vi "Intake Controller.vi"(8 "error in":errorcluster) -> ()   [LabVIEW 2019]
doc: "This VI executes continuously carrying out the current operation and responding to updates or new operations. It will often contain the timing or control code that is difficult to place directly in TeleOp. This VI generally opens all sensors and motors and isolates the rest of the robot code from knowing how the operations are carried out."
uses:
  <vilib>/Rock Robotics/WPI/Framework/Completion Status.ctl
  Intake Setpoints.ctl
  Intake Operations.ctl
  <vilib>/Rock Robotics/WPI/ThirdParty/REV Robotics/SPARK MAX/Typedef/Spark MAX Idle Mode.ctl
  <vilib>/Rock Robotics/WPI/ThirdParty/REV Robotics/SPARK MAX/Typedef/Spark MAX Control Type.ctl
  <vilib>/Rock Robotics/Network Tables/NT Write Boolean.vi
panel:
  out "Sensor Position":dbl
  out "up/down chart":T1(graph)
  in  "PID Constants":T2={"P Gain"=0.0325, "I Gain"=0.0, "D Gain"=0.0, "F Gain"=0.0, "I Zone"=0.0, "Min Output"=-0.3, "Max Output"=1.0}
  in  "Interactive Values":T3
  out "Current\nCmd":string
  in  "Buttons":cluster{"Execute Cmd":bool, "Abort Cmd":bool}
  out "Command Timing":cluster{"Start Time (ms)":u32, "Iterations":i32}
  out "Status":T5
  # "Tip: It may be helpful to observe inputs and sensor values.\nYou may also want to display tuning or debugging controls."
  # "Interactive Command: You may fill in the settings for a command\nand schedule it with the Execute button. You can observe and abort\nany command while fine tuning the code for the controller."
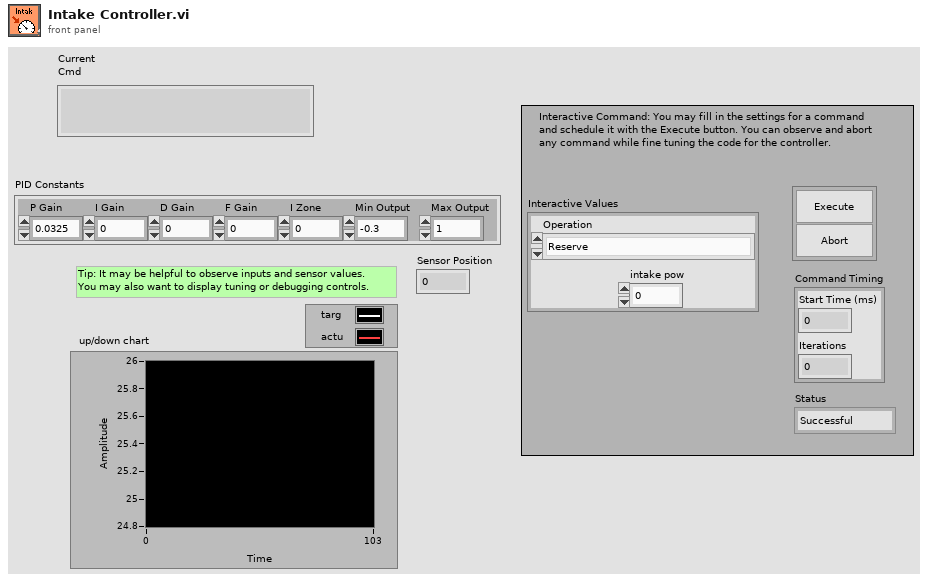
[diagram p1: front panel]
types:
  T1 = cluster{"intake down value":dbl, "Sensor Position":dbl}
  T2 = cluster{"P Gain":dbl, "I Gain":dbl, "D Gain":dbl, "F Gain":dbl, "I Zone":dbl, "Min Output":dbl, "Max Output":dbl}
  T3 = typedef "Intake Setpoints.ctl" = cluster{"Operation":T4, "intake pow":dbl}
  T4 = typedef "Intake Operations.ctl" = enum16{"Reserve", "Read Current", "Immediate"}
  T5 = typedef "Completion Status.ctl" = enum16{"Successful", "Aborted", "Incomplete"}
  T6 = typedef "Spark MAX Idle Mode.ctl" = enum16{"Coast", "Brake"}
  T7 = typedef "WPI_MotorControlDeviceRef.ctl" = cluster{"DeviceStatus":errorcluster, "Type":T8, "PWM":cluster{"PWM Channel":T9, "DeadBand":T10}, "CAN":cluster{"Device Number":u8, "SetOutput VI Ref":variant, "GetOutput VI Ref":variant, "Enable VI Ref":variant, "Disable VI Ref":variant, "Data":variant}, "Invert":bool, "DIO PWM":cluster{"PWM \"Enable\" Channel":T9, "DIOChannel":T11, "PWM Rate":dbl}}
  T8 = typedef "WPI_MotorControlType.ctl" = enum16{"PWM", "CAN", "DIO PWM"}
  T9 = typedef "FPGA_DIOPWMChannel.ctl" = enum8{"PWM 0", "PWM 1", "PWM 2", "PWM 3", "PWM 4", "PWM 5", "PWM 6", "PWM 7", "PWM 8", "PWM 9", "PWM MXP 0", "PWM MXP 1", "PWM MXP 2", "PWM MXP 3", "PWM MXP 4", "PWM MXP 5", "PWM MXP 6", "PWM MXP 7", "PWM MXP 8", "PWM MXP 9", "Invalid"}
  T10 = typedef "WPI_PWMDeadband.ctl" = cluster{"Name":string, "maxPositivePwm":i32, "minPositivePwm":i32, "centerPwm":i32, "maxNegativePwm":i32, "minNegativePwm":i32, "angularRange":u16}
  T11 = typedef "FPGA_DIOChannel.ctl" = enum8{"DIO 0", "DIO 1", "DIO 2", "DIO 3", "DIO 4", "DIO 5", "DIO 6", "DIO 7", "DIO 8", "DIO 9", "DIO MXP 0", "DIO MXP 1", "DIO MXP 2", "DIO MXP 3", "DIO MXP 4", "DIO MXP 5", "DIO MXP 6", "DIO MXP 7", "DIO MXP 8", "DIO MXP 9", "DIO MXP 10", "DIO MXP 11", "DIO MXP 12", "DIO MXP 13", "DIO MXP 14", "DIO MXP 15", "SPI Port CS1", "SPI Port CS2", "SPI Port CS3", "SPI Port MISO", "SPI Port MOSI", "Invalid"}
  T12 = typedef "Command Status Info.ctl" = cluster{"Name":string, "Status":T5, "notifier out":T13}
  T13 = typedef "Completion Notifier.ctl" = refnum<notifier>
  T14 = cluster{"Current Command":T3, "Command Timing":cluster{"Start Time (ms)":u32, "Iterations":i32}, "Command Arguments":cluster{"Command Info":T12, "Description":string, "Default Command":T3, "queue out":refnum<queue>, "Subsystem Name":string}}
  T15 = typedef "Spark MAX Control Type.ctl" = enum16{"Percent VBus", "Voltage", "Velocity", "Position", "Smart Motion", "Current", "Smart Velocity"}
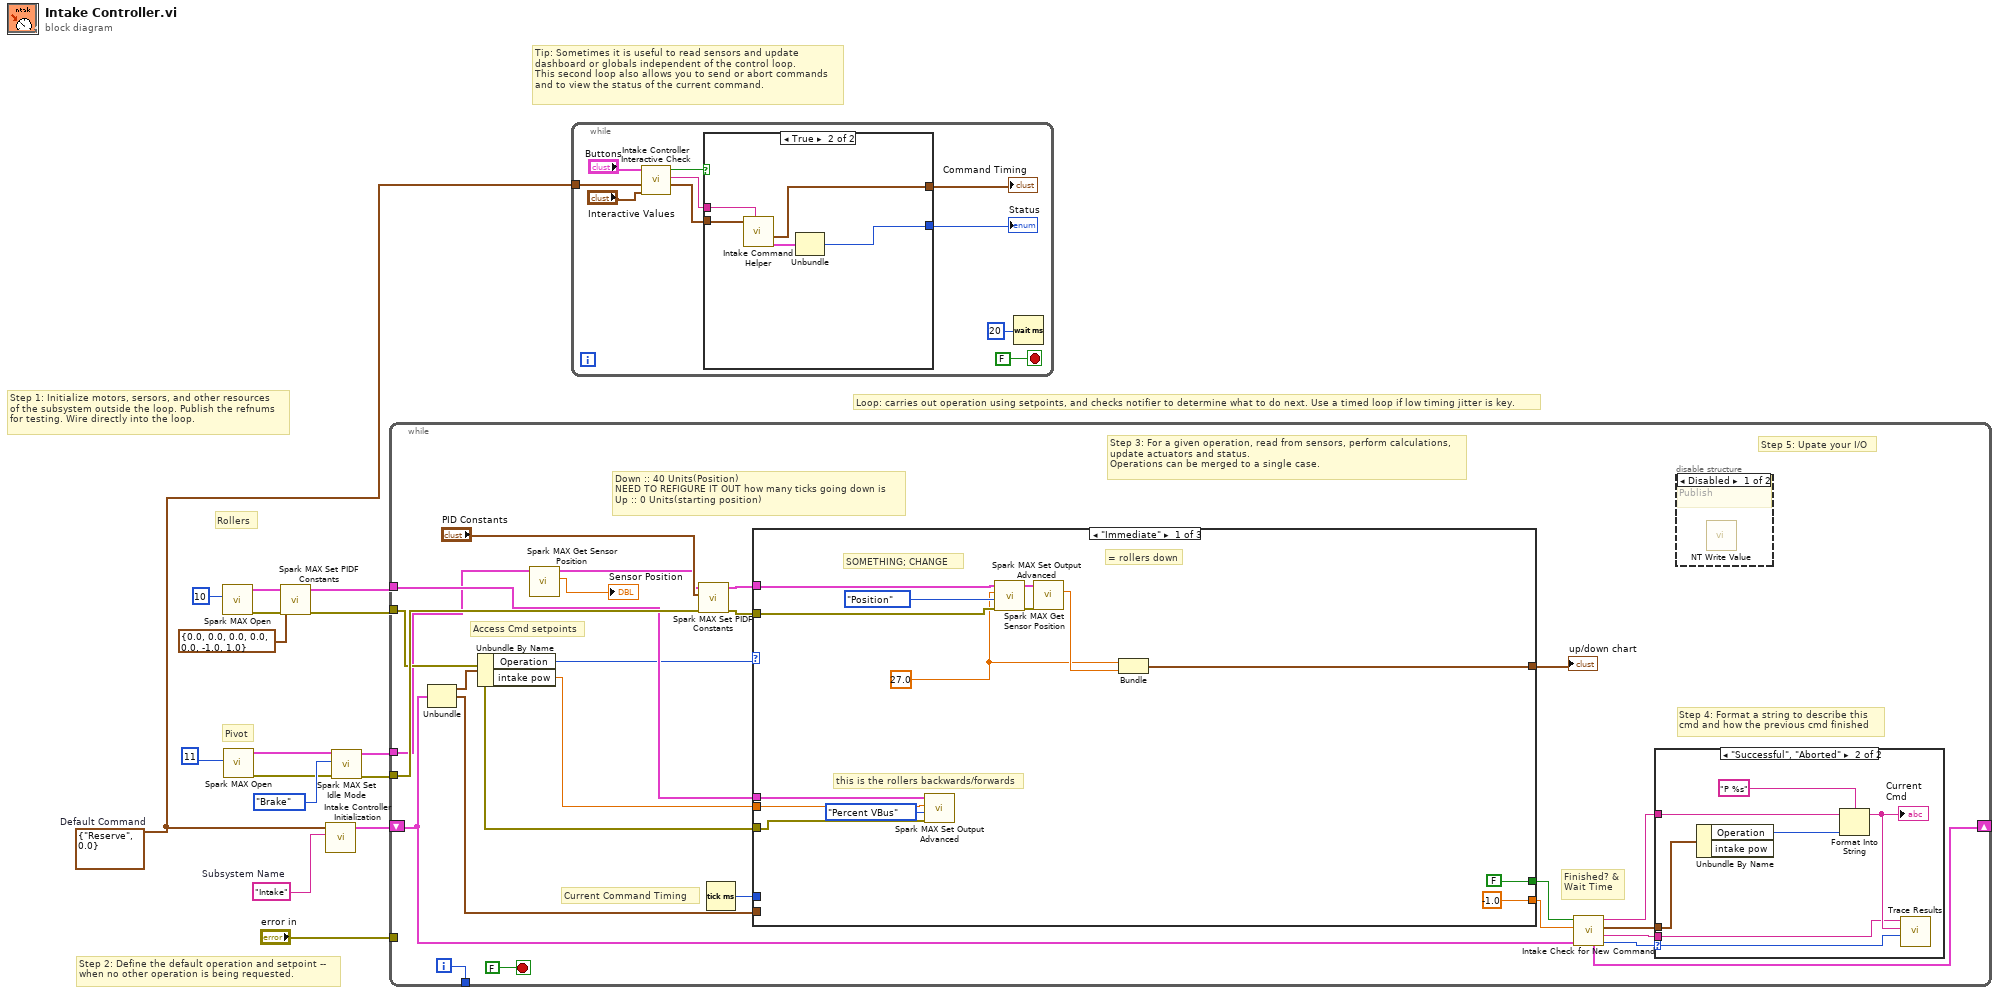
[diagram p0: block diagram]
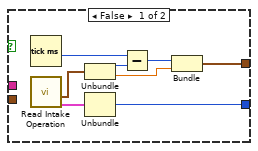
[diagram p2: hidden frame]
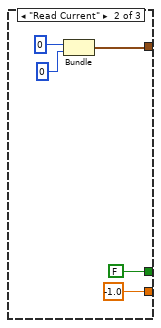
[diagram p5: hidden frame]
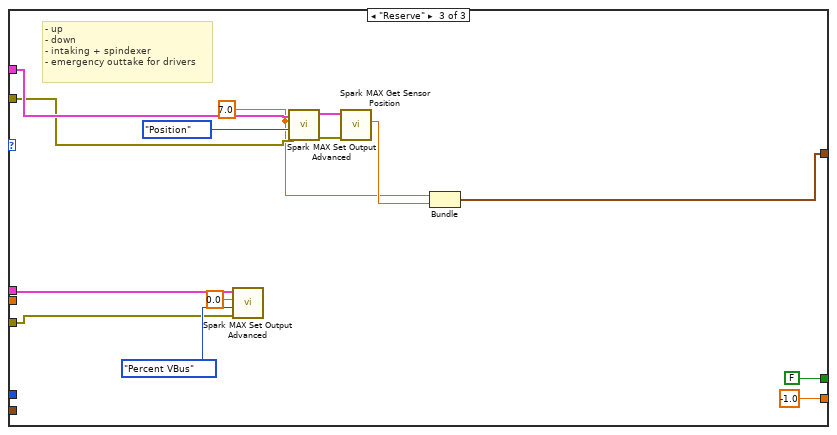
[diagram p6: hidden frame]
diagram:
  w13 = T3 {"Operation"=enum."Reserve", "intake pow"=0.0}  # Default Command
  w14 = "Intake"  # Subsystem Name
  # "Pivot"
  # "Rollers"
  # "Tip: Sometimes it is useful to read sensors and update\ndashboard or globals independent of the control loop.\nThis second loop also allows you to send or abort commands\nand to view the status of the current command."
  # "Step 2: Define the default operation and setpoint --\nwhen no other operation is being requested."
  # "Step 1: Initialize motors, sersors, and other resources\nof the subsystem outside the loop. Publish the refnums\nfor testing. Wire directly into the loop."
  # "Loop: carries out operation using setpoints, and checks notifier to determine what to do next. Use a timed loop if low timing jitter is key."
  n1 = call <vilib>:"Spark MAX Open.vi"("Device Number"=u8 10) -> ("error out"=w4:errorcluster, "MotorControlDeviceRef"=w5:T7)  [unwired: 9 in]
  n2 = call <vilib>:"Spark MAX Open.vi"("Device Number"=u8 11) -> ("error out"=w8:errorcluster, "MotorControlDeviceRef"=w9:T7)  [unwired: 9 in]
  n3 = call <vilib>:"Spark MAX Set PIDF Constants.vi"("error in"=w4, "PID Constants"=T2 {"P Gain"=0.0, "I Gain"=0.0, "D Gain"=0.0, "F Gain"=0.0, "I Zone"=0.0, "Min Output"=-1.0, "Max Output"=1.0}, "MotorControlDeviceRef"=w5) -> ("error out"=w2:errorcluster, "MotorControlDeviceRef"=w3:T7)  [unwired: 7 in]
  n4 = call "Intake Controller Initialization.vi"("Subsystem Name"=w14, "Default Command"=w13) -> ("Current Command"=w15:T14)  [unwired: 9 in]
  n5 = call <vilib>:"Spark MAX Set Idle Mode.vi"("error in (no error)"=w8, "Idle Mode"=Spark_MAX_Idle_Mode."Brake", "MotorControlDeviceRef in"=w9) -> ("error out"=w7:errorcluster, "MotorControlDeviceRef out"=w6:T7)  [unwired: 7 in]
  n6 = while {
    shift-right: [w36] -> _
    shift-left: w15 -> [w29]
    tunnel: [w40] -> _
    tunnel: "error in" -> [_]
    tunnel: w2 -> [w24]
    tunnel: w6 -> [w19]
    tunnel: w7 -> [w26]
    tunnel: w3 -> [w25]
    i -> [w40]
    stop <- FALSE stop-if-true
    # "Down :: 40 Units(Position)\nNEED TO REFIGURE IT OUT how many ticks going down is\nUp :: 0 Units(starting position)"
    # "Step 5: Upate your I/O"
    # "Step 4: Format a string to describe this\ncmd and how the previous cmd finished"
    # "Current Command Timing"
    # "Access Cmd setpoints"
    # "Finished? &\nWait Time"
    # "Step 3: For a given operation, read from sensors, perform calculations,\nupdate actuators and status.\nOperations can be merged to a single case."
    n7 = Unbundle(w29) -> ("Current Command"=w39:T3, "Command Timing"=w37:cluster{"Start Time (ms)":u32, "Iterations":i32})  [unwired: 1 out]
    n8 = Unbundle By Name(w39) -> ("Operation"=w23:T4, "intake pow"=w22:dbl)
    n9 = call <vilib>:"Spark MAX Get Sensor Position.vi"("MotorControlDevRef in"=w19) -> ("Sensor Position"=→"Sensor Position":dbl, "MotorControlDevRef out"=w18:T7)  [unwired: 7 in, 2 out]
    n10 = call <vilib>:"Spark MAX Set PIDF Constants.vi"("error in"=w26, "PID Constants"="PID Constants", "MotorControlDeviceRef"=w18) -> ("error out"=w27:errorcluster, "MotorControlDeviceRef"=w28:T7)  [unwired: 7 in]
    n11 = Tick Count (ms)() -> (millisecond timer value=w38:u32)
    n12 = case shown="\"Immediate\"" w23 {
      tunnel: [-1.0 ("Infinite") -1.0 ("Infinite") -1.0 ("Infinite")] -> w34
      tunnel: [FALSE ("ignore previous (F)") FALSE ("ignore previous (F)") FALSE ("ignore previous (F)")] -> w35
      tunnel: w37 -> [_ _ _]
      tunnel: w38 -> [_ _ _]
      tunnel: w28 -> [w54 _ w75]
      tunnel: w27 -> [w53 _ w74]
      tunnel: w25 -> [w59 _ w71]
      tunnel: w24 -> [w58 _ w70]
      tunnel: w22 -> [w57 _ _]
      tunnel: [w55 w64 w68] -> w21
      frame "Immediate" {
        w51 = 27.0 ("intake down value")
        # "this is the rollers backwards/forwards"
        # "SOMETHING; CHANGE"
        # "= rollers down"
        n13 = call <vilib>:"Spark MAX Set Output Advanced.vi"("error in (no error)"=w58, "Control Mode"=Spark_MAX_Control_Type."Percent VBus", "Setpoint"=w57, "MotorControlDevRef"=w59) -> ()  [unwired: 6 in, 2 out]
        n14 = call <vilib>:"Spark MAX Set Output Advanced.vi"("error in (no error)"=w53, "Control Mode"=Spark_MAX_Control_Type."Position", "Setpoint"=w51, "MotorControlDevRef"=w54) -> ("error out"=w49:errorcluster, "MotorControlDevRef"=w50:T7)  [unwired: 6 in]
        n15 = call <vilib>:"Spark MAX Get Sensor Position.vi"("error in (no error)"=w49, "MotorControlDevRef in"=w50) -> ("Sensor Position"=w60:dbl)  [unwired: 6 in, 3 out]
        n16 = Bundle("intake down value"=w51, "Sensor Position"=w60) -> (w55:T1)  [unwired: 1 in]
      }
      frame "Read Current" {
        n17 = Bundle(0, 0) -> (w64:cluster{i32, i32})  [unwired: 1 in]
      }
      frame "Reserve" {
        w73 = 7.0 ("Setpoint")
        # "- up\n- down\n- intaking + spindexer\n- emergency outtake for drivers"
        n18 = call <vilib>:"Spark MAX Set Output Advanced.vi"("error in (no error)"=w70, "Control Mode"=Spark_MAX_Control_Type."Percent VBus", "Setpoint"=0.0, "MotorControlDevRef"=w71) -> ()  [unwired: 6 in, 2 out]
        n19 = call <vilib>:"Spark MAX Set Output Advanced.vi"("error in (no error)"=w74, "Control Mode"=Spark_MAX_Control_Type."Position", "Setpoint"=w73, "MotorControlDevRef"=w75) -> ("error out"=w78:errorcluster, "MotorControlDevRef"=w77:T7)  [unwired: 6 in]
        n20 = call <vilib>:"Spark MAX Get Sensor Position.vi"("error in (no error)"=w78, "MotorControlDevRef in"=w77) -> ("Sensor Position"=w79:dbl)  [unwired: 6 in, 3 out]
        n21 = Bundle("Setpoint"=w73, "Sensor Position"=w79) -> (w68:cluster{"Setpoint":dbl, "Sensor Position":dbl})  [unwired: 1 in]
      }
    }
    "up/down chart" <- w21
    n22 = call "Intake Check for New Command.vi"("Current Command"=w29, "Wait time (ms)"=w34, "Finished?"=w35) -> ("Completion"=w30:T5, "Subsystem Name"=w31:string, "Current Command"=w32:T3, "Initial Trace String"=w33:string, "NextCommand"=w36:T14)  [unwired: 4 in]
    n23 = case shown="\"Successful\", \"Aborted\"" w30 {
      selector: w30 -> [_ w48]
      tunnel: w33 -> [_ w44]
      tunnel: w32 -> [_ w45]
      tunnel: w31 -> [_ w42]
      frame "Incomplete", Default {
        # "Continuing current command"
      }
      frame "Successful", "Aborted" {
        # "Report and setup for next command"
        n24 = Unbundle By Name(w45) -> ("Operation"=w47:T4)  [unwired: 1 out]
        n25 = Format Into String(format string="P %s", initial string=w44, w47) -> (resulting string=w43:string)  [unwired: 1 in, 1 out]
        "Current\nCmd" <- w43
        n26 = call <vilib>:"Trace Results.vi"("Status of previous command"=w48, "Description"=w43, "Subsystem"=w42) -> ()  [unwired: 9 in]
      }
    }
    n27 = disable-structure shown="Disabled" {
      frame Disabled {
        # "Publish"
        n28 = call-poly <vilib>:"NT Write Value.vi"() -> ()  [unwired: 11 in, 1 out]
      }
      frame Enabled {
      }
    }
  }
  n29 = while {
    tunnel: w13 -> [w88]
    stop <- FALSE stop-if-true
    n30 = call "Intake Controller Interactive Check.vi"("Interactive Command in"="Interactive Values", "Default Command"=w88, "Buttons"="Buttons") -> ("Interactive Command out"=w85:T3, "Trace String"=w86:string, "Schedule"=w87:bool)  [unwired: 6 in]
    n31 = case shown="True" w87 {
      tunnel: [w99 w104] -> w84
      tunnel: w85 -> [_ w102]
      tunnel: [w95 w100] -> w83
      tunnel: w86 -> [_ w103]
      frame False {
        n32 = Tick Count (ms)() -> (millisecond timer value=w94:u32)
        n33 = call "Read Intake Operation.vi"() -> ("Command Info"=w92:T12, "SubSystem Data"=w93:T3)  [unwired: 9 in, 1 out]
        n34 = Unbundle(w93) -> ("Operation"=w98:T4, "intake pow"=w96:dbl)
        n35 = Unbundle(w92) -> ("Status"=w99:T5)  [unwired: 2 out]
        n36 = Subtract(x=w94, y=w98) -> (x-y=w97:u32)
        n37 = Bundle(w97, "intake pow"=w96) -> (w95:cluster{u32, "intake pow":dbl})  [unwired: 1 in]
      }
      frame True {
        n38 = call "Intake Command Helper.vi"("Description"=w103, "SubSystem Data"=w102) -> ("Command Info Out"=w101:T12, "Command Timing"=w100:cluster{"Start Time (ms)":u32, "Iterations":i32})  [unwired: 7 in, 1 out]
        n39 = Unbundle(w101) -> ("Status"=w104:T5)  [unwired: 2 out]
      }
    }
    "Status" <- w84
    "Command Timing" <- w83
    n40 = Wait (ms)(milliseconds to wait=u32 20) -> ()  [unwired: 1 out]
  }
